vi "myRIO_BRig_RT_dataMTrig_Laser_N.vi"() -> (2 "output_Laser_N":i32)   [LabVIEW 2014]
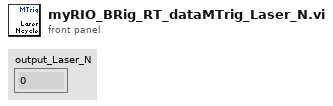
[diagram p1: front panel]
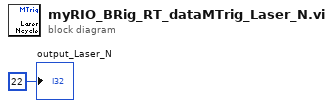
[diagram p0: block diagram]
diagram:
  "output_Laser_N" <- 22 ("output_iBlock")
